vi "abortTestSeries.vi"() -> ()   [LabVIEW 2015]
panel:
  in  "AbortTestSeries":bool
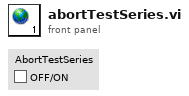
[diagram p1: front panel]
diagram:
